vi "Get Compiled Settings.vi"(8 "error in":errorcluster, 10 "Settings.Compiled":T1 {"IncomingRegisters.Settings"."Register"."Data Type" format="%.0x"; "IncomingRegisters.Refs"."Refs"."Data Reference" format="%.0x"; "OutgoingRegisters.Settings"."Register"."Data Type" format="%.0x"; "OutgoingRegisters.Refs"."Refs"."Data Reference" format="%.0x"; "IncomingDMA.Settings"."Data Type" format="%.0x"; "IncomingDMA.Settings"."DMA.Settings"."DMA Host Buffer" items=["1 Second"=1, "2 Seconds"=2, "5 Seconds"=5, "10 Seconds"=10]; "IncomingDMA.Settings"."DMA.Settings"."dt" format="%#_p"; "IncomingDMA.Settings"."DMA.Settings"."Update Rate" items=["1 Hz"=1, "2 Hz"=2, "5 Hz"=5, "10 Hz"=10]; "OutgoingDMA.Settings"."Data Type" format="%.0x"; "OutgoingDMA.Settings"."DMA.Settings"."DMA Host Buffer" items=["1 Second"=1, "2 Seconds"=2, "5 Seconds"=5, "10 Seconds"=10]; "OutgoingDMA.Settings"."DMA.Settings"."dt" format="%#_p"; "OutgoingDMA.Settings"."DMA.Settings"."Update Rate" items=["1 Hz"=1, "2 Hz"=2, "5 Hz"=5, "10 Hz"=10]}, 11 "VS Engine in":refnum<class "VS Engine.lvclass">) -> (0 "error out":errorcluster, 2 "data":T1 {"IncomingRegisters.Settings"."Register"."Data Type" format="%.0x"; "IncomingRegisters.Refs"."Refs"."Data Reference" format="%.0x"; "OutgoingRegisters.Settings"."Register"."Data Type" format="%.0x"; "OutgoingRegisters.Refs"."Refs"."Data Reference" format="%.0x"; "IncomingDMA.Settings"."Data Type" format="%.0x"; "IncomingDMA.Settings"."DMA.Settings"."DMA Host Buffer" items=["1 Second"=1, "2 Seconds"=2, "5 Seconds"=5, "10 Seconds"=10]; "IncomingDMA.Settings"."DMA.Settings"."dt" format="%#_p"; "IncomingDMA.Settings"."DMA.Settings"."Update Rate" items=["1 Hz"=1, "2 Hz"=2, "5 Hz"=5, "10 Hz"=10]; "OutgoingDMA.Settings"."Data Type" format="%.0x"; "OutgoingDMA.Settings"."DMA.Settings"."DMA Host Buffer" items=["1 Second"=1, "2 Seconds"=2, "5 Seconds"=5, "10 Seconds"=10]; "OutgoingDMA.Settings"."DMA.Settings"."dt" format="%#_p"; "OutgoingDMA.Settings"."DMA.Settings"."Update Rate" items=["1 Hz"=1, "2 Hz"=2, "5 Hz"=5, "10 Hz"=10]}, 3 "VS Engine out":refnum<class "VS Engine.lvclass">)   [LabVIEW 2024, in "VS Engine Abstraction.lvlib" / "VS Engine.lvclass"]
uses:
  VS Engine.lvclass
  VS Engine.lvclass/VS Engine.ctl
  Addon Shared/SubVIs/Constants.vi
  Addon Shared/FPGA Addon Shared.lvlib
  <vilib>/NI VeriStand/Custom Device API/Custom Device API.lvlib
  <vilib>/NI VeriStand/Custom Device API/Get Item Property (Variant).vi
  Addon Shared/Types/Delacing Scheme.ctl
  Addon Shared/Types/DMA Acquisition Mode.ctl
  Addon Shared/Types/DMA Settings.ctl
  <vilib>/NI VeriStand/Custom Device API/Waveform Data Reference.ctl
  Addon Shared/Types/FPGA Addon Data Type.ctl
  Addon Shared/Types/Compiled.DMASettings.ctl
  <vilib>/NI VeriStand/Custom Device API/Data Reference.ctl
  <vilib>/NI VeriStand/Custom Device API/Block Data Reference.ctl
  Addon Shared/Types/Scalar Type.ctl
  Addon Shared/Types/Register Information.ctl
  Addon Shared/Types/Compiled.RegisterSettings.ctl
  Addon Shared/Types/FPGA Settings.ctl
  <vilib>/NI VeriStand/Custom Device API/Custom Device Target Type.ctl
  Addon Shared/Types/Compiled.Settings.ctl
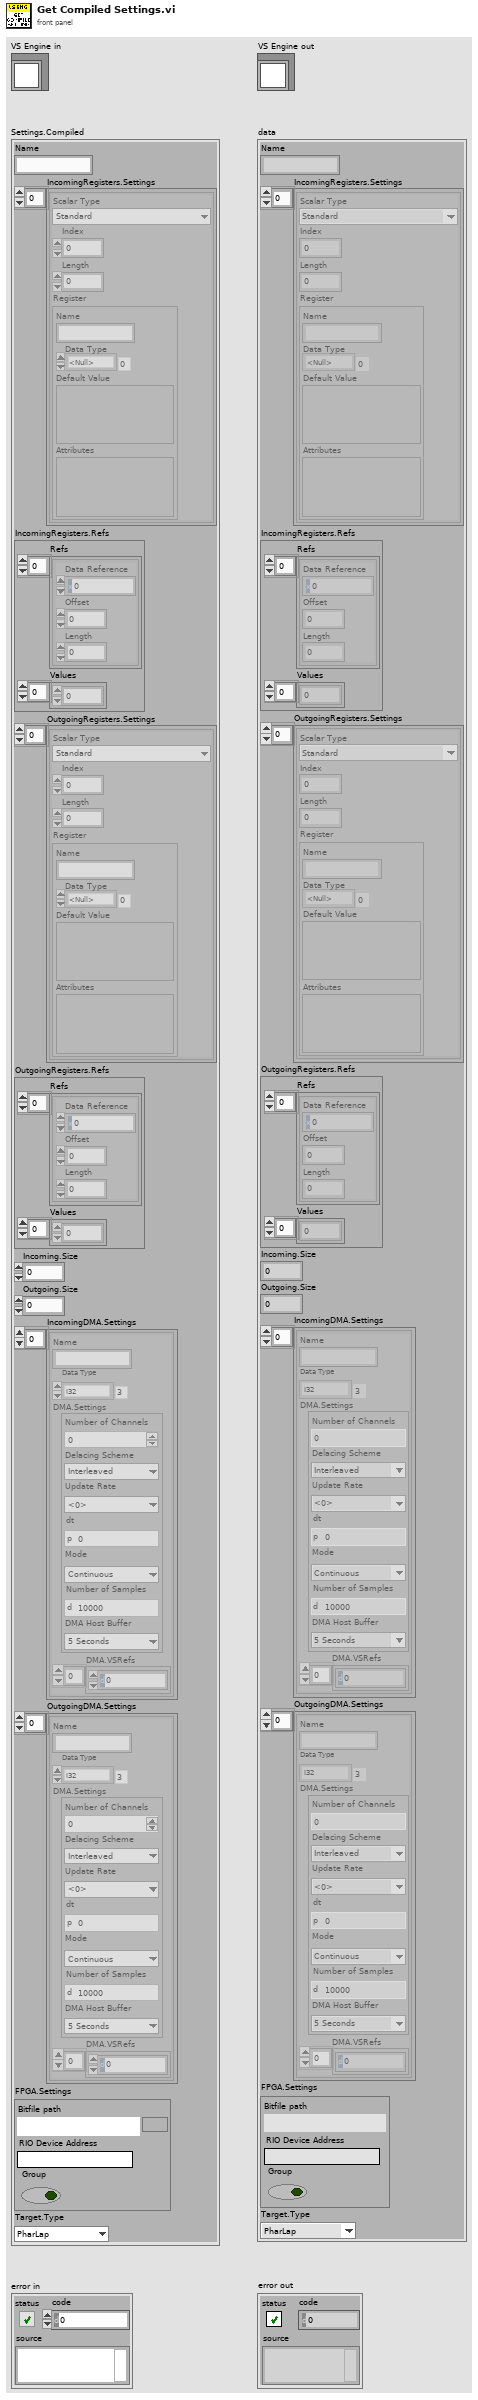
[diagram p1: front panel]
types:
  T1 = typedef "FPGA Addon Shared.lvlib/Compiled.Settings.ctl" = cluster{"Name":string, "IncomingRegisters.Settings":T2[], "IncomingRegisters.Refs":cluster{"Refs":T6[], "Values":dbl[]}, "OutgoingRegisters.Settings":T2[], "OutgoingRegisters.Refs":cluster{"Refs":T6[], "Values":dbl[]}, "Incoming.Size":i32, "Outgoing.Size":i32, "IncomingDMA.Settings":T8[], "OutgoingDMA.Settings":T8[], "FPGA.Settings":T13, "Target.Type":T14}
  T2 = typedef "FPGA Addon Shared.lvlib/Compiled.RegisterSettings.ctl" = cluster{"Scalar Type":T3, "Index":i32, "Length":i32, "Register":T4}
  T3 = typedef "FPGA Addon Shared.lvlib/Scalar Type.ctl" = enum16{"Standard", "Bitpacked"}
  T4 = typedef "FPGA Addon Shared.lvlib/Register Information.ctl" = cluster{"Name":string, "Data Type":T5, "Default Value":variant, "Attributes":variant}
  T5 = typedef "FPGA Addon Shared.lvlib/FPGA Addon Data Type.ctl" = enum8{"<Null>", "I8", "I16", "I32", "I64", "U8", "U16", "U32", "U64", "SGL", "Boolean", "Analog PWM In Settings", "Analog PWM In", "Digital PWM In Settings", "Digital PWM In", "Digital PWM Out", "Sine Out", "FXP", "FXP+/-24.5", "FXP+/-16.5", "FXP+/-32.8", "FXP+/-64.32", "FXP+/-16.7", "FXP+/-20.5", "FXP+/-27.5", "FXP+/-32.16", "FXP+16.3", "FXP+18.3", "Digital Static In", "Digital Static Out", "Digital Static In Settings", "Digital WSS Out", "Quad Encoder Settings", "Quad Encoder In", "Group"}
  T6 = typedef "Custom Device API.lvlib/Block Data Reference.ctl" = cluster{"Data Reference":T7, "Offset":u64, "Length":u64}
  T7 = typedef "Custom Device API.lvlib/Data Reference.ctl" = i32
  T8 = typedef "FPGA Addon Shared.lvlib/Compiled.DMASettings.ctl" = cluster{"Name":string, "Data Type":T5, "DMA.Settings":T9, "DMA.VSRefs":T12[]}
  T9 = typedef "FPGA Addon Shared.lvlib/DMA Settings.ctl" = cluster{"Number of Channels":u8, "Delacing Scheme":T10, "Update Rate":u32, "dt":dbl, "Mode":T11, "Number of Samples":u32, "DMA Host Buffer":u32}
  T10 = typedef "FPGA Addon Shared.lvlib/Delacing Scheme.ctl" = enum8{"Interleaved", "Bitpacked"}
  T11 = typedef "FPGA Addon Shared.lvlib/DMA Acquisition Mode.ctl" = enum8{"Continuous", "Triggered Finite"}
  T12 = typedef "Custom Device API.lvlib/Waveform Data Reference.ctl" = i32
  T13 = typedef "FPGA Addon Shared.lvlib/FPGA Settings.ctl" = cluster{"Bitfile path":path, "RIO Device Address":string, "Group":bool}
  T14 = typedef "Custom Device API.lvlib/Custom Device Target Type.ctl" = enum16{"PharLap", "VxWorks", "Windows", "Linux_32_ARM", "Linux_x64"}
  T15 = typedef "Custom Device API.lvlib/Custom Device Item Ref.ctl" = u64
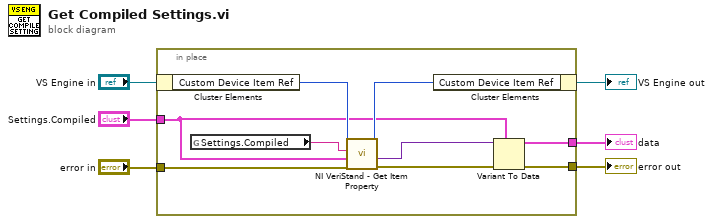
[diagram p0: block diagram]
diagram:
  n1 = in-place {
    in-place-border: [w15] -> w6
    in-place-border: [w10] -> w4
    in-place-border: "Settings.Compiled" -> [w7]
    in-place-border: "error in" -> [w14]
    n2 = in-place-cluster #1("VS Engine in") -> ("Custom Device Item Ref"=w9:T15)
    n3 = global read "Constants.vi" "Settings.Compiled"() -> (w12:string)
    n4 = call-poly <vilib>:"NI VeriStand - Get Item Property.vi"("error in (no error)"=w14, "Default Value"=w7, "Property Name"=w12, "Item Ref in"=w9) -> ("error out"=w13:errorcluster, "Value"=w11:variant, "Item Ref out"=w8:T15)  [unwired: 4 in, 1 out]
    n5 = in-place-cluster #1("Custom Device Item Ref"=w8) -> (→"VS Engine out":refnum<class "VS Engine.lvclass">)
    n6 = Variant To Data(error in=w13, type=w7, Variant=w11) -> (data=w10:T1, error out=w15:errorcluster)
  }
  "error out" <- w6
  "data" <- w4
